vi "GetObjectID.vi"(0 "reference in":refnum<class "G#Object.lvclass">, 5 "error in (no error)":errorcluster) -> (14 "reference out":refnum<class "G#Object.lvclass">, 15 "object ID":u32 format="%x", 19 "error out":errorcluster)   [LabVIEW 2017, in "G#Object.lvclass"]
doc: "Returns the unique object ID for the specified object."
uses:
  G#Object.lvclass
  G#Object.lvclass/G#Object.ctl
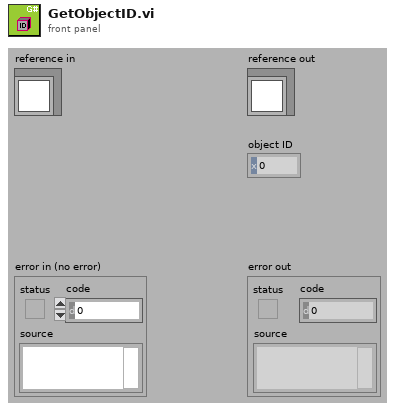
[diagram p1: front panel]
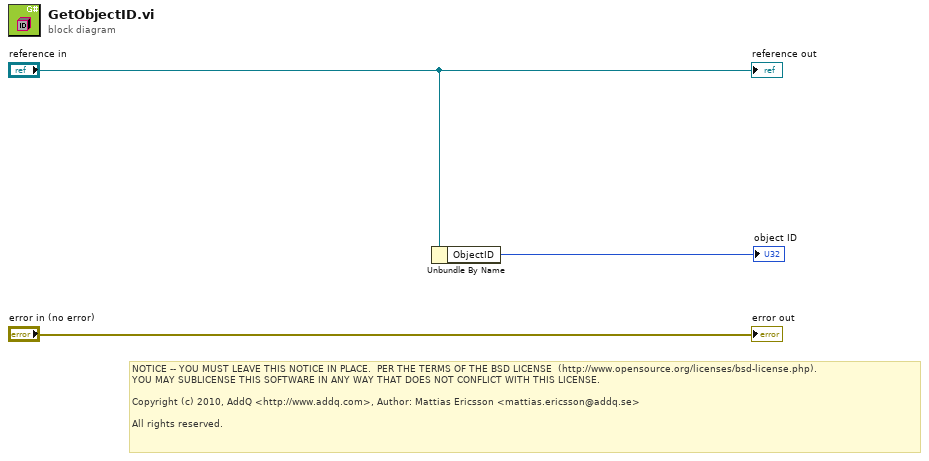
[diagram p0: block diagram]
diagram:
  # "NOTICE -- YOU MUST LEAVE THIS NOTICE IN PLACE.  PER THE TERMS OF THE BSD LICENSE  (http://www.opensource.org/licenses/bsd-license.php).\nYOU MAY SUBLICENSE THIS SOFTWARE IN ANY WAY THAT DOES NOT CONFLICT WITH THIS LICENSE.\n\nCopyright (c) 2010, AddQ <http://www.addq.com>, Author: Mattias Ericsson <mattias.ericsson@addq.se>\n\nAll rights reserved."
  n1 = Unbundle By Name("reference in") -> ("ObjectID"=→"object ID":u32)
  "error out" <- "error in (no error)"
  "reference out" <- "reference in"
